vi "programaprincipal.vi"() -> ()   [LabVIEW 2019]
uses:
  <vilib>/addons/control/pid/pid.llb/PID (DBL).vi
  <vilib>/addons/control/pid/NI_PID_pid.lvlib
panel:
  in  "Retardo":dbl
  out "Grafica":cluster{"Y":dbl, "U":dbl}(graph)
  in  "Lazo cerrado":bool
  in  "Set point":dbl
  out "den":string
  out "num":string
  out "n":i32
  out "Y":dbl format="%.2f"
  in  "Entrada\nescalon":dbl
  in  "Dt":dbl
  in  "Den":dbl[](array[numeric])
  in  "Num":dbl[](array[numeric])
  # "Y(S)"
  # "="
  # "U(S)"
  # "Lazo abierto"
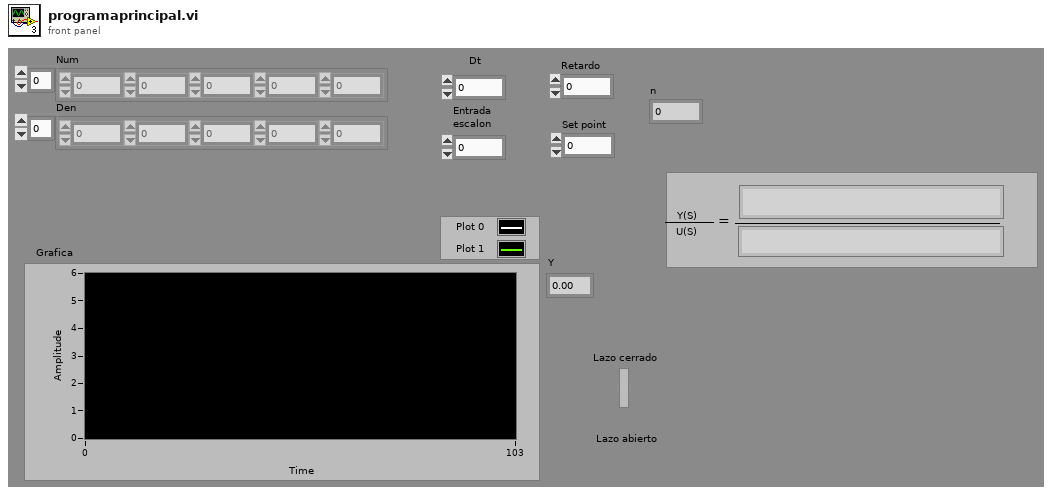
[diagram p1: front panel]
types:
  T1 = cluster{"proportional gain (Kc)":dbl, "integral time (Ti, min)":dbl, "derivative time (Td, min)":dbl}
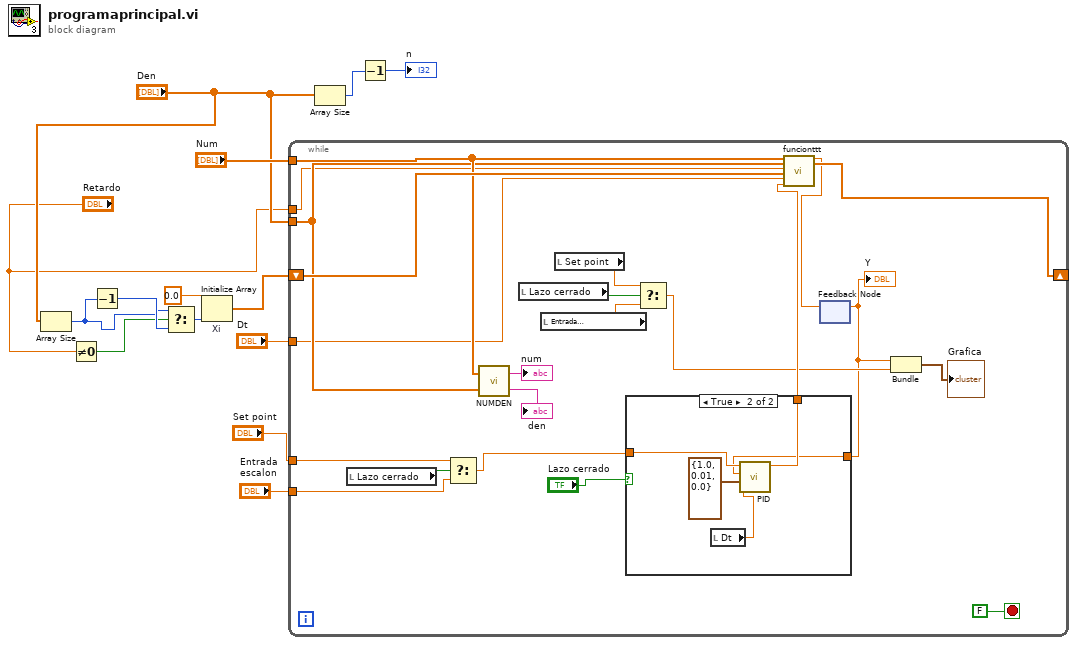
[diagram p0: block diagram]
diagram:
  n1 = Array Size(array="Den") -> (size(s)=w3:i32)
  n2 = Not Equal To 0?(x="Retardo") -> (x != 0?=w2:bool)
  n3 = Decrement(x=w3) -> (x-1=w4:i32)
  n4 = Select(t=w3, s=w2, f=w4) -> (s? t:f=w1:i32)
  n5 = Initialize Array "Xi"(0.0 ("element"), w1) -> (w12:dbl[])
  n6 = while {
    tunnel: "Num" -> [w34]
    tunnel: "Den" -> [w33]
    shift-right: [w25] -> _
    shift-left: w12 -> [w36]
    tunnel: "Dt" -> [w16]
    tunnel: "Set point" -> [w30]
    tunnel: "Entrada\nescalon" -> [w29]
    tunnel: "Retardo" -> [w15]
    stop <- FALSE stop-if-true
    n7 = local read "Lazo cerrado"() -> (w27:bool)
    n8 = Select(t=w30, s=w27, f=w29) -> (s? t:f=w24:dbl)
    n9 = call "NUMDEN.vi"("DENOMINADOR"=w33, "NUMERADOR"=w34) -> ("den"=→"den":string, "num"=→"num":string)
    n10 = local read "Lazo cerrado"() -> (w20:bool)
    n11 = local read "Entrada\nescalon"() -> (w22:dbl)
    n12 = local read "Set point"() -> (w21:dbl)
    n13 = Select(t=w21, s=w20, f=w22) -> (s? t:f=w19:dbl)
    n14 = feedback #1() -> (w18:dbl)  [unwired: 1 in]
    "Y" <- w18
    n15 = case shown="True" "Lazo cerrado" {
      tunnel: w24 -> [w37 w40]
      tunnel: [w37 w39] -> w26
      tunnel: w18 -> [_ w38]
      frame False {
      }
      frame True {
        n16 = local read "Dt"() -> (w42:dbl)
        n17 = call-poly <vilib>:"PID.vi"("dt (s)"=w42, "PID gains"=T1 {"proportional gain (Kc)"=1.0, "integral time (Ti, min)"=0.01, "derivative time (Td, min)"=0.0}, "process variable"=w38, "setpoint"=w40) -> ("output"=w39:dbl)  [unwired: 6 in, 1 out]
      }
    }
    n18 = call "funcionttt.vi"("Num"=w34, "Den"=w33, "Retardo"=w15, "XINIT"=w36, "DT"=w16, "U"=w26) -> ("Y"=w23:dbl, "Out"=w25:dbl[])  [unwired: 12 in]
    n19 = feedback-in #1(w23) -> ()
    n20 = Bundle("Y"=w18, "Entrada\nescalon"=w19) -> (→"Grafica":cluster{"Y":dbl, "Entrada\nescalon":dbl})  [unwired: 1 in]
  }
  n21 = Array Size(array="Den") -> (size(s)=w10:i32)
  n22 = Decrement(x=w10) -> (x-1=→"n":i32)
